vi "New VI.vi"() -> ()   [LabVIEW 2016]
panel:
  in  "Boolean 3":bool
  in  "Boolean 2":bool
  in  "Boolean":bool
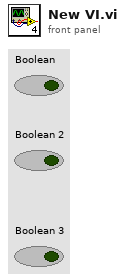
[diagram p1: front panel]
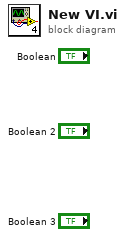
[diagram p0: block diagram]
diagram:
